vi "Power Limiter.vi"(9 "MRequested":dbl, 10 "bIMotorCalculated":bool, 11 "IBattery's":dbl) -> (2 "MOutput":dbl format="%.2f")   [LabVIEW 2015]
uses:
  Global Data.vi
  <vilib>/addons/control/pid/pid.llb/PID (DBL).vi
  <vilib>/addons/control/pid/NI_PID_pid.lvlib
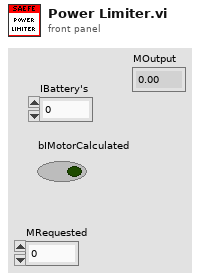
[diagram p1: front panel]
types:
  T1 = cluster{"proportional gain (Kc)":dbl, "integral time (Ti, min)":dbl, "derivative time (Td, min)":dbl}
  T2 = typedef "MC Voltage.ctl" = cluster{"VMCPhaseAB":dbl, "VMCPhaseBC":dbl, "VMCOutput":dbl, "VMCBattery":dbl}
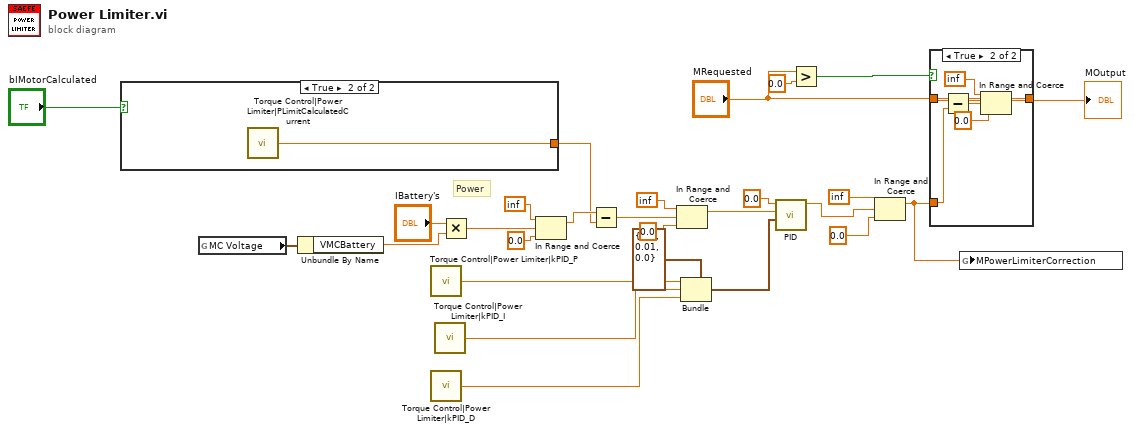
[diagram p0: block diagram]
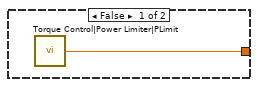
[diagram p3: hidden frame]
diagram:
  # "Power"
  n1 = case shown="True" "bIMotorCalculated" {
    tunnel: [w28 w29] -> w3
    frame False {
      n2 = call "Torque Control|Power Limiter|PLimit"() -> ("Value"=w28:sgl)
    }
    frame True {
      n3 = call "Torque Control|Power Limiter|PLimitCalculatedCurrent"() -> ("Value"=w29:sgl)
    }
  }
  n4 = global read "Global Data.vi" "MC Voltage"() -> (w25:T2)
  n5 = Unbundle By Name(w25) -> ("VMCBattery"=w27:dbl)
  n6 = call "Torque Control|Power Limiter|kPID_P"() -> ("Value"=w19:sgl)
  n7 = call "Torque Control|Power Limiter|kPID_D"() -> ("Value"=w17:sgl)
  n8 = call "Torque Control|Power Limiter|kPID_I"() -> ("Value"=w18:sgl)
  n9 = Multiply(x="IBattery's", y=w27) -> (x*y=w14:dbl)
  n10 = In Range and Coerce(upper limit=inf, x=w14, lower limit=0.0) -> (coerced(x)=w4:dbl)  [unwired: 1 out]
  n11 = Subtract(x=w4, y=w3) -> (x-y=w22:dbl)
  n12 = In Range and Coerce(upper limit=inf, x=w22, lower limit=0.0 ("upper limit")) -> (coerced(x)=w21:dbl)  [unwired: 1 out]
  n13 = Bundle(cluster=T1 {"proportional gain (Kc)"=1.0, "integral time (Ti, min)"=0.01, "derivative time (Td, min)"=0.0} ("PID gains"), "proportional gain (Kc)"=w19, "integral time (Ti, min)"=w18, "derivative time (Td, min)"=w17) -> (w16:T1)
  n14 = call-poly <vilib>:"PID.vi"("PID gains"=w16, "process variable"=w21, "setpoint"=0.0) -> ("output"=w8:dbl)  [unwired: 7 in, 1 out]
  n15 = Greater?(x="MRequested", y=0.0) -> (0:w10:bool)
  n16 = In Range and Coerce(upper limit=inf, x=w8, lower limit=0.0 ("setpoint")) -> (coerced(x)=w7:dbl)  [unwired: 1 out]
  n17 = case shown="True" w10 {
    tunnel: w7 -> [_ w36]
    tunnel: [w30 w31] -> w15
    tunnel: "MRequested" -> [w30 w35]
    frame False {
    }
    frame True {
      n18 = Subtract(x=w35, y=w36) -> (x-y=w34:dbl)
      n19 = In Range and Coerce(upper limit=inf, x=w34, lower limit=0.0) -> (coerced(x)=w31:dbl)  [unwired: 1 out]
    }
  }
  "MOutput" <- w15
  n20 = global write "Global Data.vi" "MPowerLimiterCorrection"(w7) -> ()
